vi "SpeedAccelDistanceM1.vi"() -> ()   [LabVIEW 2015]
uses:
  <instrlib>/Ion Motion Roboclaw/Ion Motion Roboclaw.lvlib
panel:
  in  "Distance":u32 max=0 step=1
  in  "Address":u8
  in  "Accel":u32(slide) max=800000 step=10000 scale=0.0..800000.0
  in  "Speed":i32(slide)=-40000 min=-40000 max=40000 step=1000 scale=-40000.0..40000.0
  out "Valid":bool
  out "error out":errorcluster
  in  "COM port":refnum<visa-resource-name>
  in  "baud rate (38400)":u32
  in  "error in (no error)":errorcluster
  # "This example assumes the Velocity PID  values have already been tuned for the motor and saved to the Roboclaw."
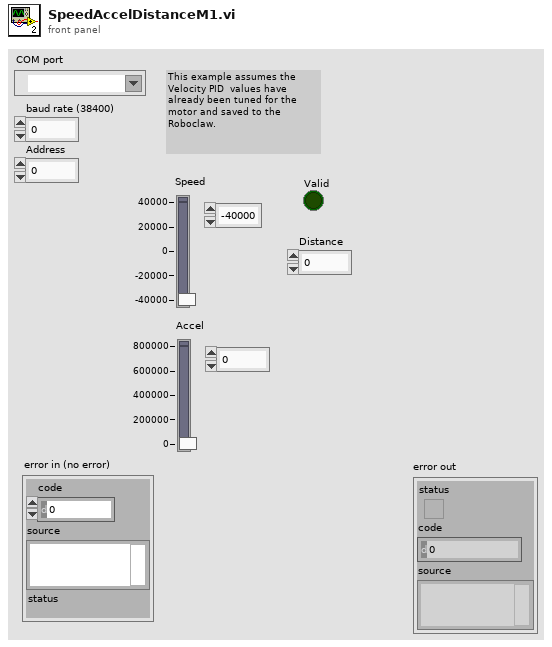
[diagram p1: front panel]
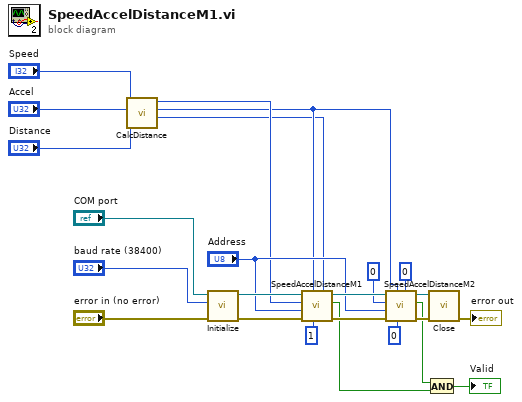
[diagram p0: block diagram]
diagram:
  n1 = call <instrlib>:"CalcDistance.vi"("Distance In"="Distance", "Accel In"="Accel", "Speed In"="Speed") -> ("Distance Out"=w1:i32, "Accel Out"=w2:u32, "Speed Out"=w3:i32)  [unwired: 6 in]
  n2 = call <instrlib>:"Initialize.vi"("error in (no error)"="error in (no error)", "baud rate (38400)"="baud rate (38400)", "COM port"="COM port") -> ("error out"=w19:errorcluster, "VISA resource name out"=w20:refnum<visa-resource-name>)  [unwired: 7 in]
  n3 = call <instrlib>:"SpeedAccelDistanceM1.vi"("Distance"=w1, "Immediate"=u8 1, "Accel"=w2, "error in (no error)"=w19, "Address"="Address", "Speed"=w3, "VISA Refnum in"=w20) -> ("error out"=w17:errorcluster, "Valid"=w7:bool, "VISA Refnum out"=w18:refnum<visa-resource-name>)  [unwired: 1 in]
  n4 = call <instrlib>:"SpeedAccelDistanceM2.vi"("Distance"=u32 0, "Immediate"=u8 0 ("Immediate 2"), "Accel"=w2, "error in (no error)"=w17, "Address"="Address", "Speed"=0 ("Speed 2"), "VISA Refnum in"=w18) -> ("error out"=w16:errorcluster, "Valid"=w8:bool, "VISA Refnum out"=w15:refnum<visa-resource-name>)  [unwired: 1 in]
  n5 = And(x=w8, y=w7) -> (x .and. y?=→"Valid":bool)
  n6 = call <instrlib>:"Close.vi"("error in (no error)"=w16, "VISA resource name"=w15) -> ("error out"=→"error out":errorcluster)  [unwired: 9 in]
